vi "writeI64.vi"(8 "error in (no error)":errorcluster, 10 "Input":i64, 11 "ModbusBuffer in":refnum<class "ModbusBufferBuilder.lvclass">) -> (0 "error out":errorcluster, 3 "ModbusBuffer out":refnum<class "ModbusBufferBuilder.lvclass">)   [LabVIEW 2016, in "ModbusBufferBuilder.lvclass"]
uses:
  ModbusBufferBuilder.lvclass
  ModbusBufferBuilder.lvclass/ModbusBufferBuilder.ctl
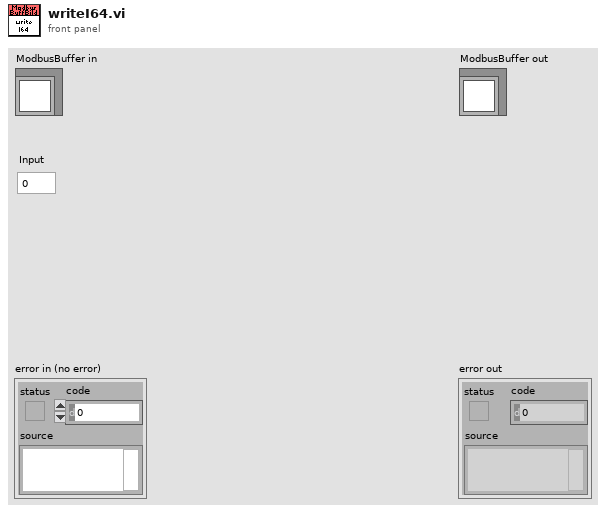
[diagram p1: front panel]
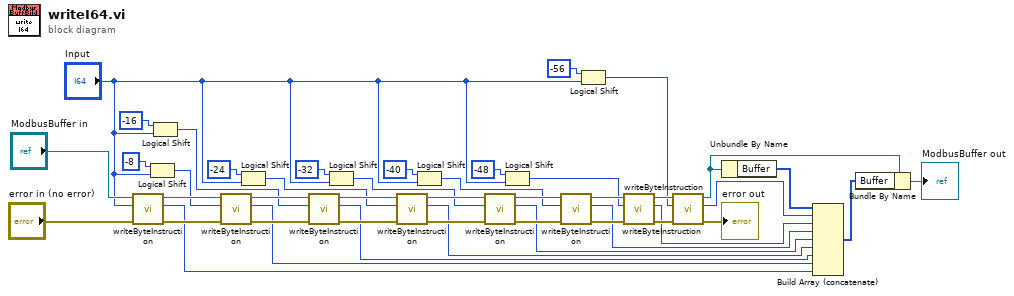
[diagram p0: block diagram]
diagram:
  n1 = call "writeByteInstruction.vi"("error in (no error)"="error in (no error)", "Input"="Input", "ModbusBuffer in"="ModbusBuffer in") -> ("error out"=w18:errorcluster, "Output"=w1:u16, "ModbusBuffer out"=w35:refnum<class "ModbusBufferBuilder.lvclass">)  [unwired: 6 in]
  n2 = Logical Shift(y=i16 -8, x="Input") -> (x << y=w26:i64)
  n3 = Logical Shift(y=i16 -16, x="Input") -> (x << y=w25:i64)
  n4 = call "writeByteInstruction.vi"("error in (no error)"=w18, "Input"=w26, "ModbusBuffer in"=w35) -> ("error out"=w17:errorcluster, "Output"=w2:u16, "ModbusBuffer out"=w34:refnum<class "ModbusBufferBuilder.lvclass">)  [unwired: 6 in]
  n5 = Logical Shift(y=i16 -24, x="Input") -> (x << y=w24:i64)
  n6 = call "writeByteInstruction.vi"("error in (no error)"=w17, "Input"=w25, "ModbusBuffer in"=w34) -> ("error out"=w16:errorcluster, "Output"=w3:u16, "ModbusBuffer out"=w33:refnum<class "ModbusBufferBuilder.lvclass">)  [unwired: 6 in]
  n7 = Logical Shift(y=i16 -32, x="Input") -> (x << y=w23:i64)
  n8 = call "writeByteInstruction.vi"("error in (no error)"=w16, "Input"=w24, "ModbusBuffer in"=w33) -> ("error out"=w15:errorcluster, "Output"=w4:u16, "ModbusBuffer out"=w32:refnum<class "ModbusBufferBuilder.lvclass">)  [unwired: 6 in]
  n9 = Logical Shift(y=i16 -40, x="Input") -> (x << y=w22:i64)
  n10 = call "writeByteInstruction.vi"("error in (no error)"=w15, "Input"=w23, "ModbusBuffer in"=w32) -> ("error out"=w14:errorcluster, "Output"=w5:u16, "ModbusBuffer out"=w31:refnum<class "ModbusBufferBuilder.lvclass">)  [unwired: 6 in]
  n11 = Logical Shift(y=i16 -48, x="Input") -> (x << y=w21:i64)
  n12 = call "writeByteInstruction.vi"("error in (no error)"=w14, "Input"=w22, "ModbusBuffer in"=w31) -> ("error out"=w13:errorcluster, "Output"=w6:u16, "ModbusBuffer out"=w30:refnum<class "ModbusBufferBuilder.lvclass">)  [unwired: 6 in]
  n13 = Logical Shift(y=i16 -56, x="Input") -> (x << y=w20:i64)
  n14 = call "writeByteInstruction.vi"("error in (no error)"=w13, "Input"=w21, "ModbusBuffer in"=w30) -> ("error out"=w12:errorcluster, "Output"=w7:u16, "ModbusBuffer out"=w29:refnum<class "ModbusBufferBuilder.lvclass">)  [unwired: 6 in]
  n15 = call "writeByteInstruction.vi"("error in (no error)"=w12, "Input"=w20, "ModbusBuffer in"=w29) -> ("error out"=→"error out":errorcluster, "Output"=w8:u16, "ModbusBuffer out"=w28:refnum<class "ModbusBufferBuilder.lvclass">)  [unwired: 6 in]
  n16 = Unbundle By Name(w28) -> ("Buffer"=w10:u16[])
  n17 = Build Array (concatenate)(w10, w8, w7, w6, w5, w4, w3, w2, w1) -> (w9:u16[])
  n18 = Bundle By Name(cluster=w28, "Buffer"=w9) -> (→"ModbusBuffer out":refnum<class "ModbusBufferBuilder.lvclass">)
